vi "OverflowOffset.vi"(3 "TPR":dbl=162.974662, 4 "Sensor Position":dbl, 5 "Current Offset":dbl) -> (1 "New Offset":dbl)   [LabVIEW 2014]
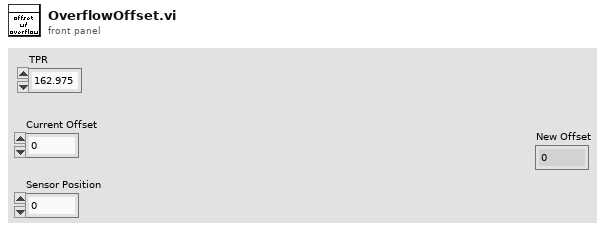
[diagram p1: front panel]
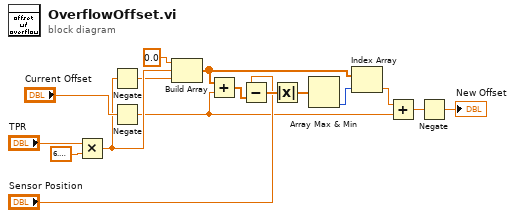
[diagram p0: block diagram]
diagram:
  n1 = Multiply(x="TPR", y=6.283185307179586) -> (x*y=w10:dbl)
  n2 = Negate(x=w10) -> (-x=w9:dbl)
  n3 = Negate(x="Current Offset") -> (-x=w1:dbl)
  n4 = Build Array(0.0 ("y"), w10, w9) -> (w6:dbl[])
  n5 = Add(x=w6, y=w1) -> (x+y=w4:dbl[])
  n6 = Subtract(x="Sensor Position", y=w4) -> (x-y=w5:dbl[])
  n7 = Absolute Value(x=w5) -> (abs(x)=w8:dbl[])
  n8 = Array Max & Min(array=w8) -> (min index (indices)=w2:i32)  [unwired: 3 out]
  n9 = Index Array(array=w6, index=w2) -> (element=w7:dbl)
  n10 = Add(x=w7, y=w1) -> (x+y=w13:dbl)
  n11 = Negate(x=w13) -> (-x=→"New Offset":dbl)
